vi "3.1.vi"() -> ()   [LabVIEW 2020]
panel:
  out "Waveform Chart 2":cluster{dbl, dbl}(graph)
  out "Array":dbl[](array[numeric])
  out "Waveform Chart":dbl[](graph)
  out "appended array":dbl[][](array[numeric])
  out "Farenheit 2":dbl[](array[numeric])
  out "min value":dbl
  out "max value":dbl
  out "Celcius rand":dbl[](array[numeric])
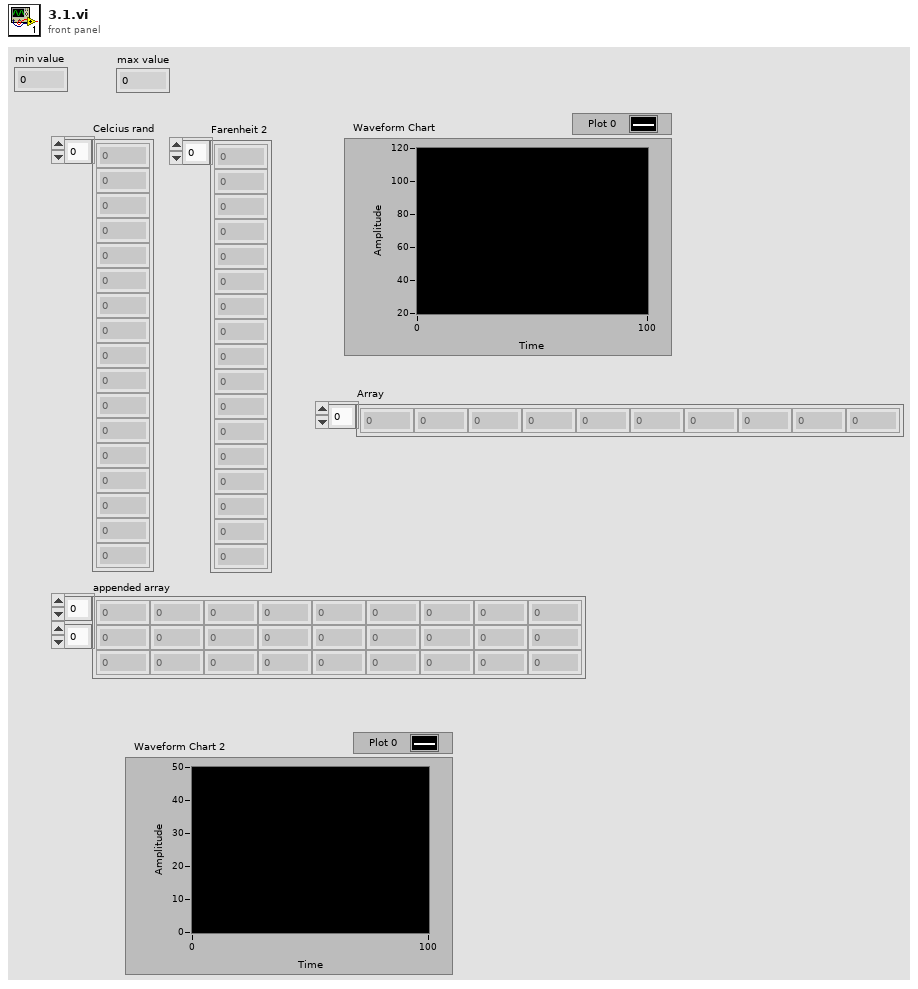
[diagram p1: front panel]
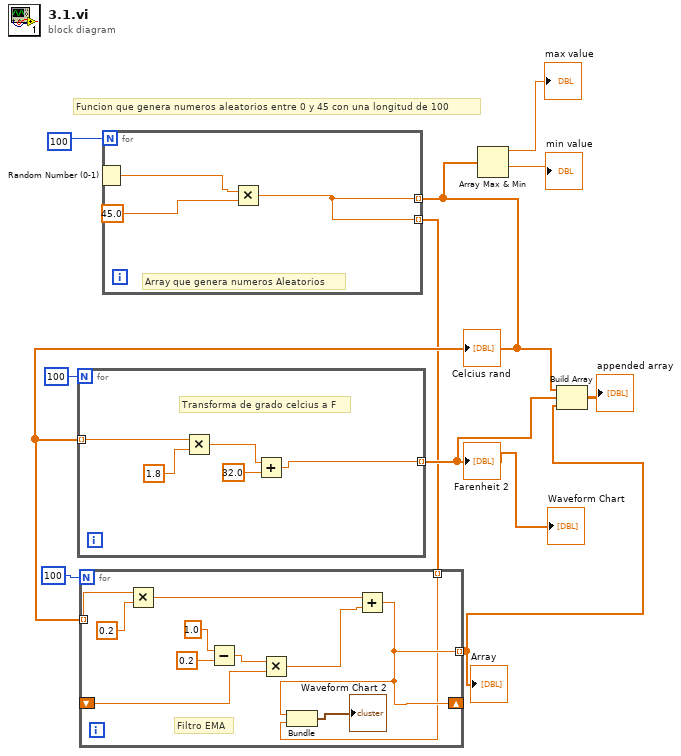
[diagram p0: block diagram]
diagram:
  # "Funcion que genera numeros aleatorios entre 0 y 45 con una longitud de 100"
  n1 = for {
    N: 100 -> [_]
    tunnel: [w11] -> w4 mode=indexing
    tunnel: [w11] -> w1 mode=indexing
    # "Array que genera numeros Aleatorios"
    n2 = Random Number (0-1)() -> (number: 0 to 1=w12:dbl)
    n3 = Multiply(x=w12, y=45.0) -> (x*y=w11:dbl)
  }
  "Celcius rand" <- w4
  n4 = for {
    N: 100 -> [_]
    tunnel: w4 -> [w18] mode=indexing
    tunnel: [w14] -> w5 mode=indexing
    # "Transforma de grado celcius a F"
    n5 = Multiply(x=w18, y=1.8) -> (x*y=w16:dbl)
    n6 = Add(x=w16, y=32.0) -> (x+y=w14:dbl)
  }
  "Farenheit 2" <- w5
  "Waveform Chart" <- w5
  n7 = for {
    N: 100 -> [_]
    tunnel: w4 -> [w29] mode=indexing
    shift-right: [w20] -> _
    shift-left: _ -> [w23]
    tunnel: [w20] -> w2 mode=indexing
    tunnel: w1 -> [w19] mode=indexing
    # "Filtro EMA"
    n8 = Multiply(x=w29, y=0.2) -> (x*y=w27:dbl)
    n9 = Subtract(x=1.0, y=0.2) -> (x-y=w24:dbl)
    n10 = Multiply(x=w24, y=w23) -> (x*y=w22:dbl)
    n11 = Add(x=w27, y=w22) -> (x+y=w20:dbl)
    n12 = Bundle(w20, w19) -> (→"Waveform Chart 2":cluster{dbl, dbl})  [unwired: 1 in]
  }
  "Array" <- w2
  n13 = Array Max & Min(array=w4) -> (max value=→"max value":dbl, min value=→"min value":dbl)  [unwired: 2 out]
  n14 = Build Array(w4, w5, w2) -> (→"appended array":dbl[][])
